vi "Check Disk Space.vi"(8 "error in":errorcluster, 11 "path":path=path "C:/Users/BOAS-USER/Documents/Data/200328 mainGUI coding") -> (0 "error out":errorcluster, 2 "Free space":dbl, 3 "Full Disk Space":dbl)   [LabVIEW 2018]
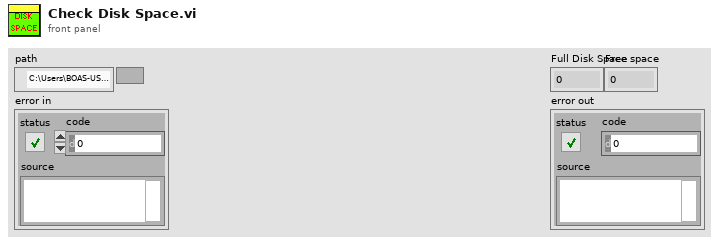
[diagram p1: front panel]
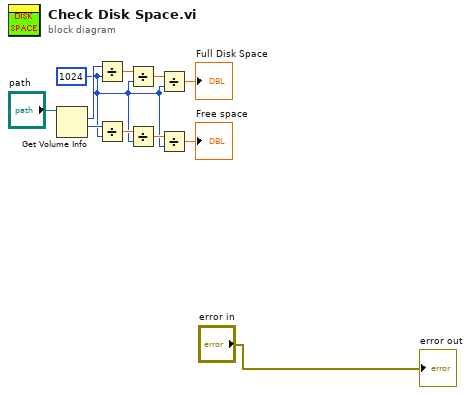
[diagram p0: block diagram]
diagram:
  w4 = i64 1024 ("y")
  n1 = Get Volume Info(11:"path") -> (1:w7:i64, 2:w10:i64)  [unwired: 1 in, 4 out]
  n2 = Divide(x=w10, y=w4) -> (x/y=w9:dbl)
  n3 = Divide(x=w7, y=w4) -> (x/y=w6:dbl)
  n4 = Divide(x=w9, y=w4) -> (x/y=w8:dbl)
  n5 = Divide(x=w6, y=w4) -> (x/y=w5:dbl)
  n6 = Divide(x=w8, y=w4) -> (x/y=→"Full Disk Space":dbl)
  n7 = Divide(x=w5, y=w4) -> (x/y=→"Free space":dbl)
  "error out" <- "error in"
